vi "Restart cRIO.vi"(8 "error in (no error)":errorcluster, 11 "File transfer":T1) -> (0 "error out":errorcluster)   [LabVIEW 2022 SP3]
uses:
  <vilib>/nisyscfg/Close (System).vi
  <vilib>/nisyscfg/nisyscfg.lvlib
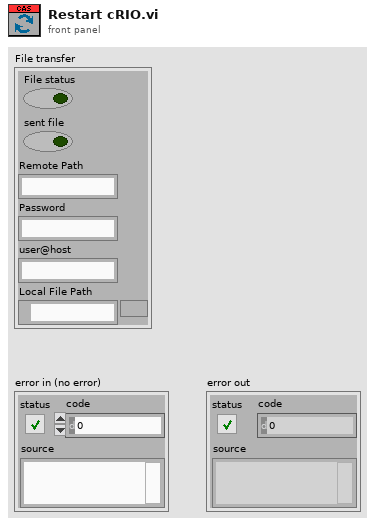
[diagram p1: front panel]
types:
  T1 = cluster{"File status":bool, "sent file":bool, "Remote Path":string, "Password":string, "user@host":string, "Local File Path":path}
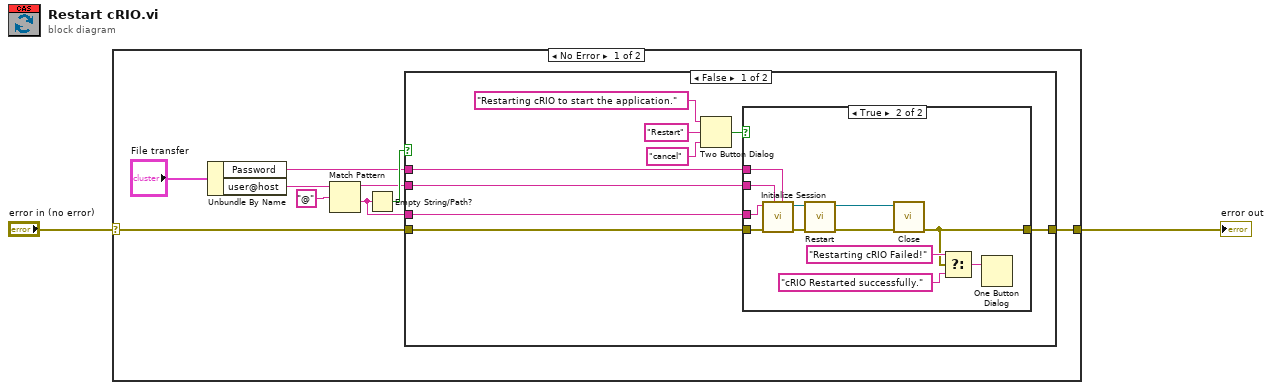
[diagram p0: block diagram]
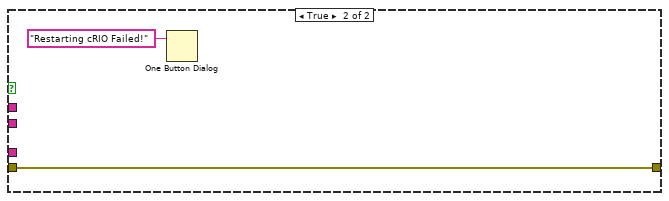
[diagram p3: hidden frame]
diagram:
  n1 = case shown="No Error" "error in (no error)" {
    selector: "error in (no error)" -> [w11 w36]
    tunnel: [w10 w36] -> w1
    frame No Error {
      n2 = Unbundle By Name("File transfer") -> ("Password"=w7:string, "user@host"=w6:string)
      n3 = Match Pattern(string=w6, regular expression="@") -> (before substring=w4:string, after substring=w3:string)  [unwired: 1 in, 2 out]
      n4 = Empty String/Path?(string/path=w3) -> (empty?=w9:bool)
      n5 = case shown="False" w9 {
        tunnel: w11 -> [w17 w35]
        tunnel: [w16 w35] -> w10
        tunnel: w7 -> [w14 _]
        tunnel: w4 -> [w13 _]
        tunnel: w3 -> [w12 _]
        frame False {
          n6 = Two Button Dialog(message="Restarting cRIO to start the application.", 1:"cancel" ("F button name (\"Cancel\")"), 2:"Restart" ("T button name (\"OK\")")) -> (T button?=w18:bool)
          n7 = case shown="True" w18 {
            tunnel: [w21 w25] -> w16
            tunnel: w17 -> [w21 w26]
            tunnel: w13 -> [_ w24]
            tunnel: w14 -> [_ w23]
            tunnel: w12 -> [_ w22]
            frame False {
            }
            frame True {
              n8 = call <vilib>:"Initialize Session.vi"("Password"=w23, "User Name"=w24, "error in (no error)"=w26, "Target (localhost)"=w22) -> ("error out"=w28:errorcluster, "Session out"=w29:refnum<k21>)  [unwired: 6 in]
              n9 = call <vilib>:"Restart.vi"("error in (no error)"=w28, "Session in"=w29) -> ("error out"=w27:errorcluster, "Session out"=w30:refnum<k21>)  [unwired: 7 in, 1 out]
              n10 = call-poly <vilib>:"Close.vi"("error in (no error)"=w27, "Session in"=w30) -> ("error out"=w25:errorcluster)  [unwired: 9 in]
              n11 = Select(t="Restarting cRIO Failed!", s=w25, f="cRIO Restarted successfully." ("message")) -> (s? t:f=w33:string)
              n12 = One Button Dialog(message=w33) -> ()  [unwired: 1 in, 1 out]
            }
          }
        }
        frame True {
          n13 = One Button Dialog(message="Restarting cRIO Failed!" ("t")) -> ()  [unwired: 1 in, 1 out]
        }
      }
    }
    frame Error {
    }
  }
  "error out" <- w1
